vi "AdaptToInputs.vi"(0 "XRef":T8, 1 "Term Types":T5, 2 "State In":T1) -> (14 "Reply":T3, 15 "Fatal Error Out":T2, 16 "State Out":T1)   [LabVIEW 2015, in "Build JSON Array.xnode"]
uses:
  Build JSON Array.xnode
  <vilib>/XNodeSupport/XNodeXNodeRef.ctl
  <vilib>/XNodeSupport/XNodeTermTypeIDPairs.ctl
  <vilib>/XNodeSupport/XNodeTermTypeIDPair.ctl
  <vilib>/XNodeSupport/XNodeType.ctl
  <vilib>/XNodeSupport/XNodeString.ctl
  State.ctl
  <vilib>/XNodeSupport/XNodeStringArray.ctl
  <vilib>/XNodeSupport/XNodeErrorCluster.ctl
  <vilib>/Utility/Data Type/NI_Data Type.lvlib
  <vilib>/XNodeSupport/NI_XNodeSupport.lvlib
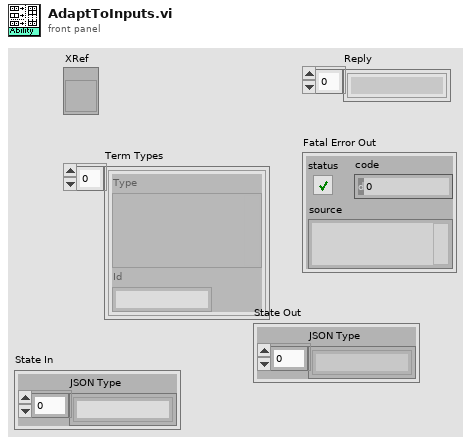
[diagram p1: front panel]
types:
  T1 = typedef "Build JSON Array.xnode/State.ctl" = cluster{"JSON Type":string[]}
  T2 = typedef "NI_XNodeSupport.lvlib/XNodeErrorCluster.ctl" = errorcluster
  T3 = typedef "NI_XNodeSupport.lvlib/XNodeStringArray.ctl" = T4[]
  T4 = typedef "NI_XNodeSupport.lvlib/XNodeString.ctl" = string
  T5 = typedef "NI_XNodeSupport.lvlib/XNodeTermTypeIDPairs.ctl" = T6[]
  T6 = typedef "NI_XNodeSupport.lvlib/XNodeTermTypeIDPair.ctl" = cluster{"Type":T7, "Id":T4}
  T7 = typedef "NI_XNodeSupport.lvlib/XNodeType.ctl" = variant
  T8 = typedef "NI_XNodeSupport.lvlib/XNodeXNodeRef.ctl" = refnum<vi>
  T9 = typedef "NI_Data Type.lvlib/Data Type.ctl" = enum8{"Invalid Type", "Void", "I8", "I16", "I32", "I64", "U8", "U16", "U32", "U64", "Single Float", "Double Float", "Extended Float", "Single Complex", "Double Complex", "Extended Complex", "Enum U8", "Enum U16", "Enum U32", "Enum U64", "Single Float With Unit", "Double Float With Unit", "Extended Float With Unit", "Single Complex with Unit", "Double Complex with Unit", "Extended Complex with Unit", "Boolean", "String", "Path", "Picture", "Tag", "Array", "Cluster", "Variant", "LV Variant", "Waveform", "Timestamp", "Digital Waveform", "Digital Data", "ExpressData", "Refnum", "External Data", "VI", "Poly VI", "LabVIEW Class Instance", "Fixed Point"}
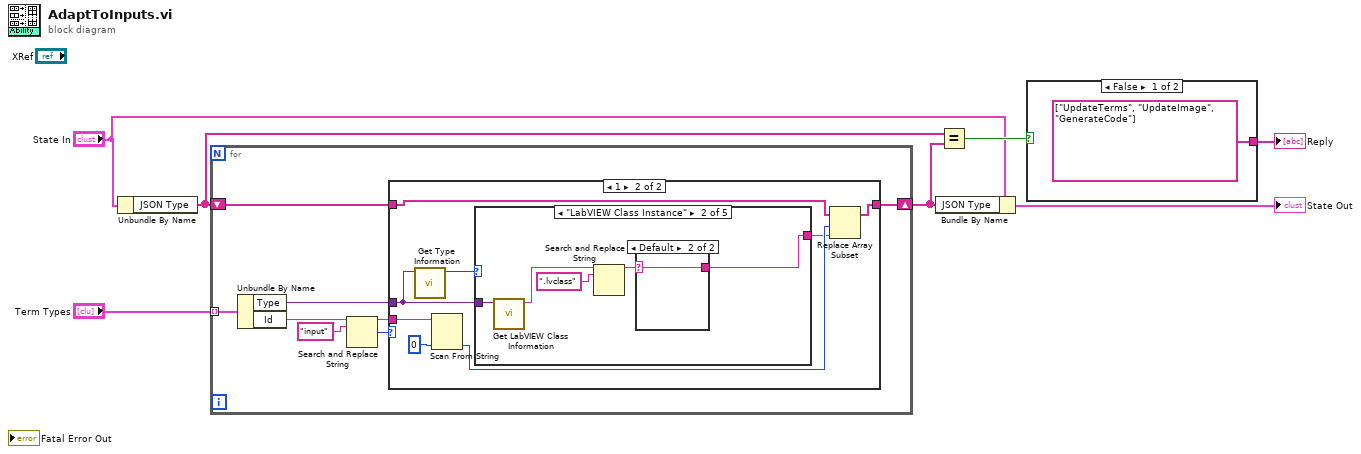
[diagram p0: block diagram]
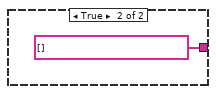
[diagram p2: hidden frame]
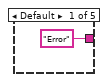
[diagram p4: hidden frame]
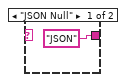
[diagram p5: hidden frame]
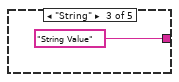
[diagram p6: hidden frame]
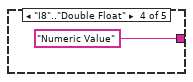
[diagram p7: hidden frame]
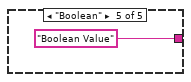
[diagram p8: hidden frame]
diagram:
  n1 = Unbundle By Name("State In") -> ("JSON Type"=w7:string[])
  n2 = for {
    tunnel: "Term Types" -> [w12] mode=indexing
    shift-right: [w8] -> w5
    shift-left: w7 -> [w10]
    n3 = Unbundle By Name(w12) -> ("Type"=w15:T7, "Id"=w14:T4)
    n4 = Search and Replace String(input string=w14, search string="input") -> (result string=w9:string, number of replacements=w11:i32)  [unwired: 6 in, 2 out]
    n5 = case shown="1" w11 {
      tunnel: w15 -> [_ w23]
      tunnel: w10 -> [w16 w20]
      tunnel: w9 -> [_ w22]
      tunnel: [w16 w17] -> w8
      frame 0, Default {
      }
      frame 1 {
        n6 = call <vilib>:"Get Type Information.vi"("Variant"=w23) -> ("Type"=w24:T9)  [unwired: 6 in, 4 out]
        n7 = Scan From String(input string=w22, default 1=0 ("default value 1")) -> (output 1=w19:i32)  [unwired: 3 in, 3 out]
        n8 = case shown="\"LabVIEW Class Instance\"" w24 {
          tunnel: w23 -> [_ w30 _ _ _]
          tunnel: ["Error" w26 "String Value" "Numeric Value" "Boolean Value"] -> w18
          frame Default {
          }
          frame "LabVIEW Class Instance" {
            n9 = call <vilib>:"Get LabVIEW Class Information.vi"("Variant"=w30) -> ("LabVIEW Class File Name"=w29:string)  [unwired: 8 in, 2 out]
            n10 = Search and Replace String(input string=w29, search string=".lvclass") -> (result string=w27:string)  [unwired: 6 in, 3 out]
            n11 = case shown="Default" w27 {
              selector: w27 -> [_ w32]
              tunnel: ["JSON" w32] -> w26
              frame "JSON Null" {
              }
              frame Default {
              }
            }
          }
          frame "String" {
          }
          frame "I8".."Double Float" {
          }
          frame "Boolean" {
          }
        }
        n12 = Replace Array Subset(array=w20, new element=w18, index=w19) -> (w17:string[])
      }
    }
  }
  n13 = Bundle By Name(cluster="State In", "JSON Type"=w5) -> (→"State Out":T1)
  n14 = Equal?(x=w7, y=w5) -> (x = y?=w6:bool)
  n15 = case shown="False" w6 {
    tunnel: [T3 ["UpdateTerms", "UpdateImage", "GenerateCode"] ("Reply") T3 [] ("Reply")] -> w1
    frame False {
    }
    frame True {
    }
  }
  "Reply" <- w1
